vi "conv.vi"(0 "Camera in":refnum<class "Camera.lvclass">, 5 "data_format":T1(ring)=enum."Mono16", 11 "error in (no error)":errorcluster) -> (4 "Camera out":refnum<class "Camera.lvclass">, 6 "conv":u64, 15 "error out":errorcluster)   [LabVIEW 2020, in "Camera.lvclass"]
doc: "Retreive the conv handle.\nThis handle allows direct access to all underlying functions of the color conversion library pco.convert."
uses:
  Camera.lvclass
  Camera.lvclass/Camera.ctl
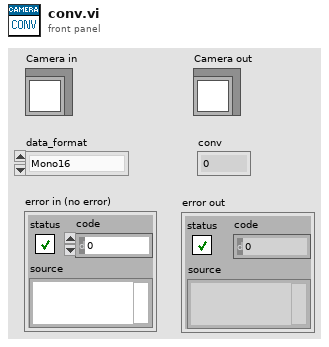
[diagram p1: front panel]
types:
  T1 = enum16{"Undefined", "Mono8", "Mono16", "BGRA8", "RGBA8", "BGRA16", "RGBA16", "CompressedMono8"}
  T2 = map{enum16{"Undefined", "Mono8", "Mono16", "BGRA8", "RGBA8", "BGRA16", "RGBA16", "CompressedMono8"}, u64}
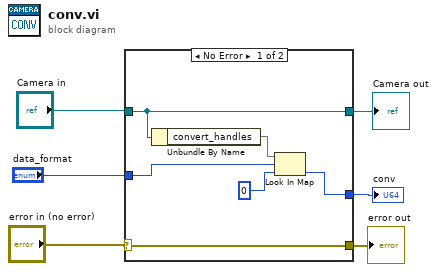
[diagram p0: block diagram]
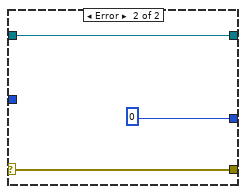
[diagram p2: hidden frame]
diagram:
  n1 = case shown="No Error" "error in (no error)" {
    selector: "error in (no error)" -> [w12 w15]
    tunnel: [w12 w15] -> w4
    tunnel: [w11 w14] -> w5
    tunnel: "Camera in" -> [w11 w14]
    tunnel: [w10 u64 0 ("dwErr")] -> w2
    tunnel: "data_format" -> [w8 _]
    frame No Error {
      n2 = Unbundle By Name(w11) -> ("convert_handles"=w9:T2)
      n3 = Look In Map(map=w9, key=w8, default value=u64 0) -> (value=w10:u64)  [unwired: 1 out]
    }
    frame Error {
    }
  }
  "error out" <- w4
  "Camera out" <- w5
  "conv" <- w2
